vi "Video feed info class VI - retrieve beginning-end cursor states.vi"(8 "error in (no error)":errorcluster, 11 "Video feed info in":refnum<class "Video feed info.lvclass">) -> (0 "error out":errorcluster, 1 "Higher Cursor value":u32, 2 "Lower Cursor value":u32, 3 "Video feed info out":refnum<class "Video feed info.lvclass">)   [LabVIEW 2010, in "Video feed info.lvclass"]
uses:
  Video feed info.lvclass
  Video feed info.lvclass/Video feed info.ctl
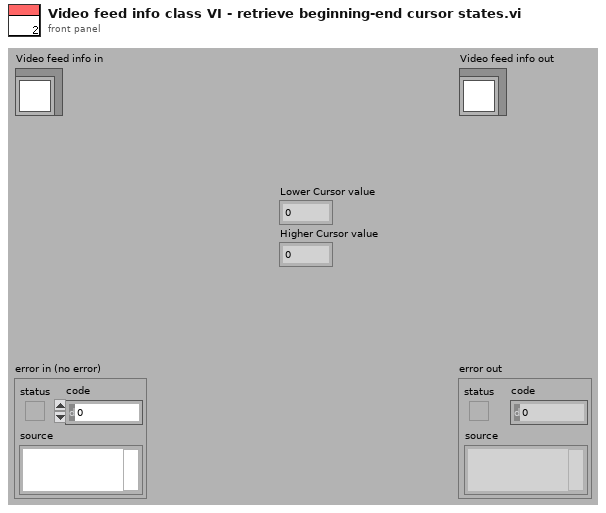
[diagram p1: front panel]
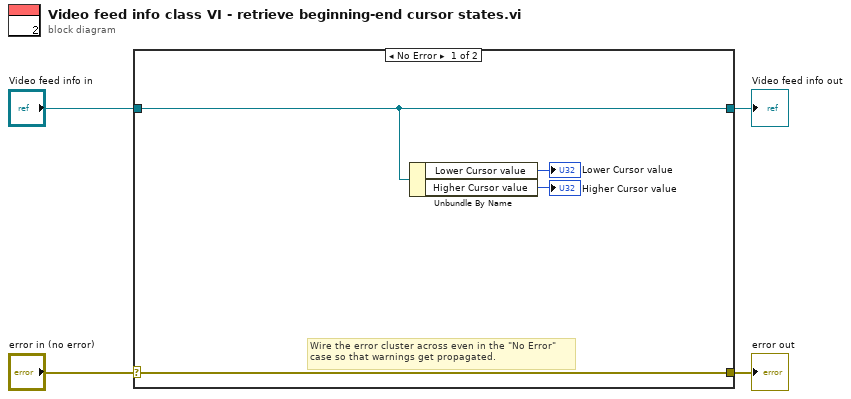
[diagram p0: block diagram]
diagram:
  n1 = case shown="No Error" "error in (no error)" {
    selector: "error in (no error)" -> [w8 w10]
    tunnel: [w8 w10] -> w3
    tunnel: [w7 w9] -> w1
    tunnel: "Video feed info in" -> [w7 w9]
    frame No Error {
      # "Wire the error cluster across even in the \"No Error\"\ncase so that warnings get propagated."
      n2 = Unbundle By Name(w7) -> ("Lower Cursor value"=→"Lower Cursor value":u32, "Higher Cursor value"=→"Higher Cursor value":u32)
    }
    frame Error {
    }
  }
  "error out" <- w3
  "Video feed info out" <- w1
